vi "Run Command.vi"(2 "Line Index In":i32, 3 "Script":string) -> (0 "Line Index Out":i32, 1 "Done":bool)   [LabVIEW 2013]
doc: "Looks at a line and runs the appropriate command. Add new commands to this vi."
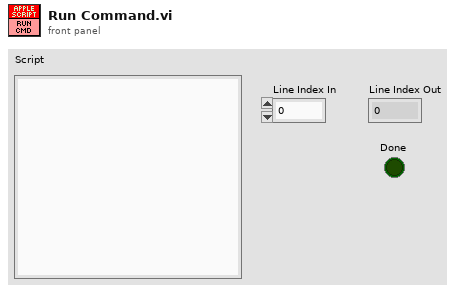
[diagram p1: front panel]
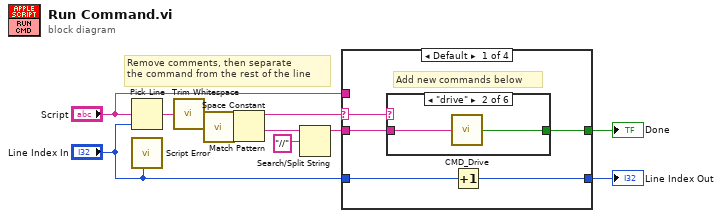
[diagram p0: block diagram]
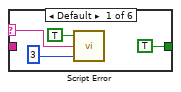
[diagram p2: hidden frame]
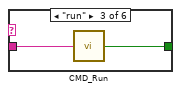
[diagram p3: hidden frame]
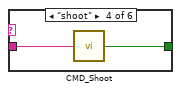
[diagram p4: hidden frame]
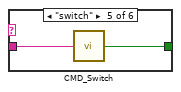
[diagram p5: hidden frame]
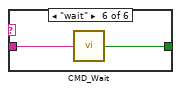
[diagram p6: hidden frame]
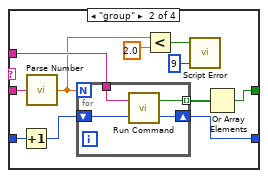
[diagram p7: hidden frame]
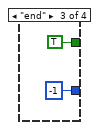
[diagram p8: hidden frame]
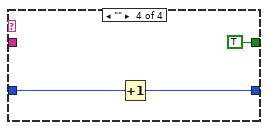
[diagram p9: hidden frame]
diagram:
  # "Remove comments, then separate\nthe command from the rest of the line"
  n1 = Pick Line(multi-line string="Script", line index="Line Index In") -> (output string=w4:string)  [unwired: 1 in]
  n2 = call "Script Error.vi"("Line Number"="Line Index In") -> ()  [unwired: 5 in]
  n3 = call <vilib>:"Trim Whitespace.vi"("string"=w4) -> ("trimmed string"=w3:string)  [unwired: 1 in]
  n4 = call <vilib>:"Space Constant.vi"() -> ("String"=w11:string)
  n5 = Match Pattern(string=w3, regular expression=w11) -> (before substring=w10:string, after substring=w5:string)  [unwired: 1 in, 2 out]
  n6 = Search/Split String(string=w5, search string/char (-)="//") -> (substring before match=w2:string)  [unwired: 1 in, 2 out]
  n7 = case shown="Default" w10 {
    selector: w10 -> [w14 _ _ _]
    tunnel: "Script" -> [_ w40 _ _]
    tunnel: "Line Index In" -> [w16 w36 _ w49]
    tunnel: [w13 w38 TRUE ("Running") TRUE ("Running")] -> w8
    tunnel: [w15 w37 -1 ("Line Index Out") w48] -> w7
    tunnel: w2 -> [w12 w41 _ _]
    frame Default {
      # "Add new commands below"
      n8 = case shown="\"drive\"" w14 {
        selector: w14 -> [w17 _ _ _ _ _]
        tunnel: [TRUE w22 w24 w25 w27 w29] -> w13
        tunnel: w12 -> [_ w21 w23 w26 w28 w30]
        frame Default {
          n9 = call "Script Error.vi"("Error?"=TRUE, "Error Details"=w17, "Error Code"=3) -> ()  [unwired: 3 in]
        }
        frame "drive" {
          n10 = call "CMD_Drive.vi"("Line"=w21) -> ("Done"=w22:bool)
        }
        frame "run" {
          n11 = call "CMD_Run.vi"("Line"=w23) -> ("Done"=w24:bool)
        }
        frame "shoot" {
          n12 = call "CMD_Shoot.vi"("Line"=w26) -> ("Done"=w25:bool)
        }
        frame "switch" {
          n13 = call "CMD_Switch.vi"("Line"=w28) -> ("Done"=w27:bool)
        }
        frame "wait" {
          n14 = call "CMD_Wait.vi"("Line"=w30) -> ("Done"=w29:bool)
        }
      }
      n15 = Increment(x=w16) -> (x+1=w15:i32)
    }
    frame "group" {
      n16 = Increment(x=w36) -> (x+1=w35:i32)
      n17 = call "Parse Number.vi"("String"=w41) -> ("Number"=w33:dbl)
      n18 = for {
        N: w33 -> [_]
        tunnel: w40 -> [w45]
        tunnel: [w44] -> w39 mode=indexing
        shift-right: [w43] -> w37
        shift-left: w35 -> [w42]
        n19 = call "Run Command.vi"("Line Index In"=w42, "Script"=w45) -> ("Line Index Out"=w43:i32, "Done"=w44:bool)
      }
      n20 = Less?(x=w33, y=2.0) -> (x < y?=w32:bool)
      n21 = call "Script Error.vi"("Error?"=w32, "Error Code"=9) -> ()  [unwired: 4 in]
      n22 = Or Array Elements(Boolean array=w39) -> (logical OR=w38:bool)
    }
    frame "end" {
    }
    frame "" {
      n23 = Increment(x=w49) -> (x+1=w48:i32)
    }
  }
  "Line Index Out" <- w7
  "Done" <- w8
